vi "BluetoothRobot.vi"() -> ()   [LabVIEW 2010]
uses:
  <vilib>/Instr/_visa.llb/VISA Configure Serial Port (Instr).vi
  <vilib>/Utility/inputDevices.llb/closeJoystick.vi
  <vilib>/Utility/inputDevices.llb/joystickAcquire.vi
panel:
  in  "baud rate (9600)":u32=115200
  in  "device index":i32=4
  in  "stop":bool
  out "Write Data":string
  in  "Write":bool
  in  "VISA resource name":refnum<visa-resource-name>="COM14"
  out "error out":errorcluster
  in  "error in (no error)":errorcluster
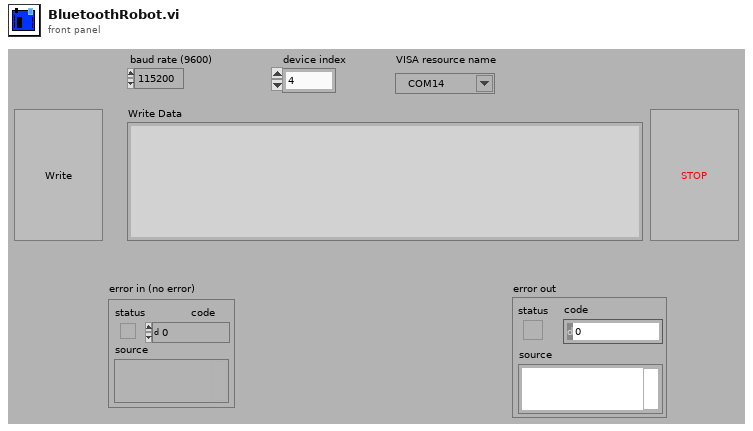
[diagram p1: front panel]
types:
  T1 = cluster{"X axis":i32, "Y axis":i32, "Z axis":i32, "X axis rotation":i32, "Y axis rotation":i32, "Z axis rotation":i32, "U axis":i32, "V axis":i32}
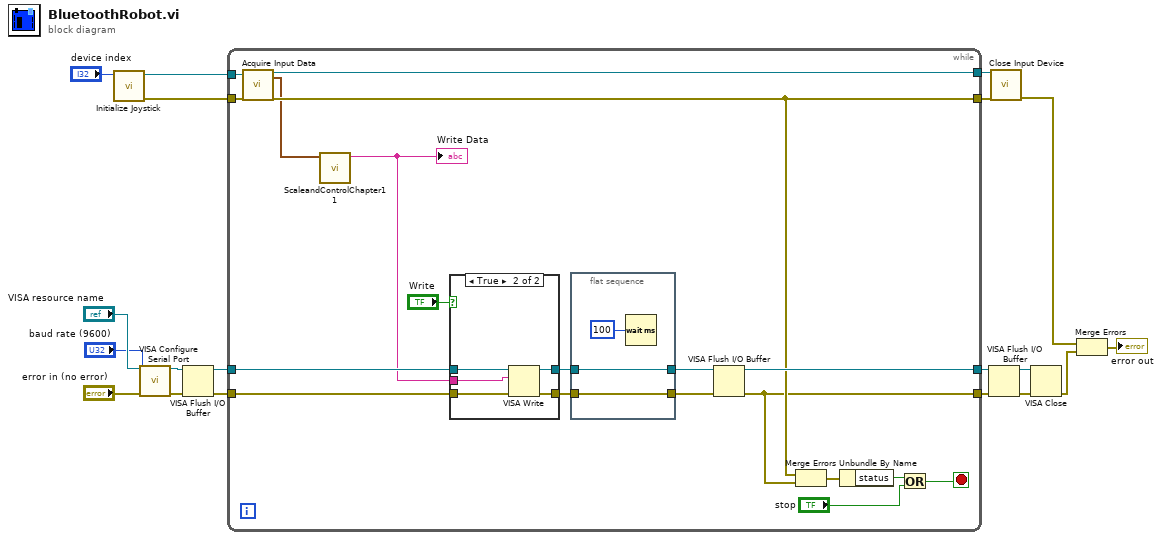
[diagram p0: block diagram]
diagram:
  n1 = call <vilib>:"Initialize Joystick.vi"("device index"="device index") -> ("error out"=w12:errorcluster, "device ID"=w13:refnum<k1>)  [unwired: 9 in]
  n2 = call-poly "VISA Configure Serial Port"("VISA resource name"="VISA resource name", "baud rate (9600)"="baud rate (9600)", "error in (no error)"="error in (no error)") -> ("VISA resource name out"=w14:refnum<visa-resource-name>, "error out"=w15:errorcluster)  [unwired: 11 in]
  n3 = VISA Flush I/O Buffer(VISA resource name=w14, error in (no error)=w15) -> (VISA resource name out=w9:refnum<visa-resource-name>, error out=w8:errorcluster)  [unwired: 1 in]
  n4 = while {
    tunnel: w13 -> [w38]
    tunnel: w12 -> [w37]
    tunnel: [w36] -> w11
    tunnel: [w23] -> w10
    tunnel: w9 -> [w29]
    tunnel: w8 -> [w28]
    tunnel: [w27] -> w7
    tunnel: [w22] -> w6
    stop <- w30 stop-if-true
    n5 = call-poly <vilib>:"Acquire Input Data.vi"("device ID"=w38, "error in (no error)"=w37) -> ("device ID"=w36:refnum<k1>, "axis info"=w21:T1, "error out"=w23:errorcluster)  [unwired: 13 in, 2 out]
    n6 = call "ScaleandControlChapter11.vi"("axis info"=w21) -> ("String"=w20:string)  [unwired: 10 in]
    "Write Data" <- w20
    n7 = case shown="True" "Write" {
      tunnel: [w43 w48] -> w34
      tunnel: [w42 w47] -> w35
      tunnel: w29 -> [w43 w46]
      tunnel: w28 -> [w42 w45]
      tunnel: w20 -> [_ w44]
      frame False {
      }
      frame True {
        n8 = VISA Write(VISA resource name=w46, write buffer=w44, error in (no error)=w45) -> (VISA resource name out=w48:refnum<visa-resource-name>, error out=w47:errorcluster)  [unwired: 1 out]
      }
    }
    n9 = flat-sequence {
      tunnel: w34 -> [w41]
      tunnel: [w41] -> w26
      tunnel: w35 -> [w40]
      tunnel: [w40] -> w25
      frame #0 {
        n10 = Wait (ms)(milliseconds to wait=u32 100) -> ()  [unwired: 1 out]
      }
    }
    n11 = VISA Flush I/O Buffer(VISA resource name=w26, error in (no error)=w25) -> (VISA resource name out=w27:refnum<visa-resource-name>, error out=w22:errorcluster)  [unwired: 1 in]
    n12 = Merge Errors(w23, w22) -> (w24:errorcluster)
    n13 = Unbundle By Name(w24) -> ("status"=w33:bool)
    n14 = Or(x=w33, y="stop") -> (x .or. y?=w30:bool)
  }
  n15 = VISA Flush I/O Buffer(VISA resource name=w7, error in (no error)=w6) -> (VISA resource name out=w16:refnum<visa-resource-name>, error out=w17:errorcluster)  [unwired: 1 in]
  n16 = call-poly <vilib>:"Close Input Device.vi"("error in (no error)"=w10, "device ID"=w11) -> ("error out"=w2:errorcluster)  [unwired: 8 in]
  n17 = VISA Close(VISA resource name=w16, error in (no error)=w17) -> (error out=w4:errorcluster)
  n18 = Merge Errors(w2, w4) -> (→"error out":errorcluster)
